vi "Traffic Control Project with Some more features.vi"() -> ()   [LabVIEW 2019]
uses:
  <vilib>/LabVIEW Interface for Arduino/Type Defs/Connection Type.ctl
  <vilib>/LabVIEW Interface for Arduino/Type Defs/Pin Mode.ctl
  <vilib>/LabVIEW Interface for Arduino/Type Defs/Board Type.ctl
  <vilib>/LabVIEW Interface for Arduino/LabVIEW Interface for Arduino.lvlib
panel:
  out "Boolean 3":bool
  out "Boolean 2":bool
  out "Boolean":bool
  in  "milliseconds to wait 3":u32
  in  "milliseconds to wait 2":u32
  in  "milliseconds to wait":u32
  in  "stop":bool
  in  "VISA resource":refnum<visa-resource-name>
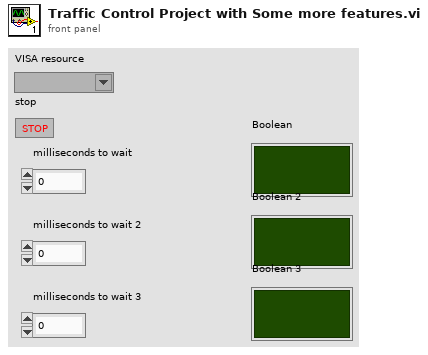
[diagram p1: front panel]
types:
  T1 = typedef "LabVIEW Interface for Arduino.lvlib/Board Type.ctl" = enum16{"Uno", "Dimuelanove w/Atmega 328", "Mega 2560"}
  T2 = typedef "LabVIEW Interface for Arduino.lvlib/Pin Mode.ctl" = enum8{"Input", "Output"}
  T3 = typedef "LabVIEW Interface for Arduino.lvlib/Connection Type.ctl" = enum8{"USB / Serial", "XBEE", "BlueSmirf (Bluetooth)"}
  T4 = typedef "LabVIEW Interface for Arduino.lvlib/Arduino Resource.ctl" = cluster{"VISA resource":refnum<visa-resource-name>, "Board Type":T1, "Connection Type":enum8{"USB / Serial"}, "Bytes Per Packet (15)":u8}
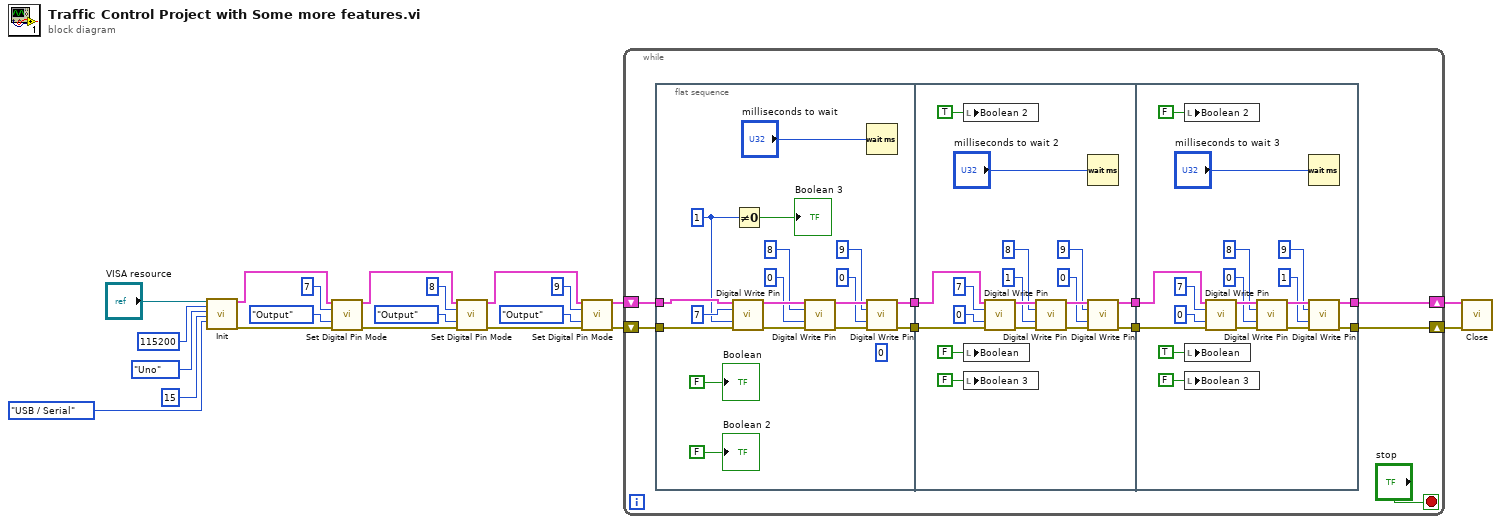
[diagram p0: block diagram]
diagram:
  n1 = call <vilib>:"Init.vi"("VISA resource"="VISA resource", "Baud Rate (115200)"=u32 115200, "Board Type (Uno)"=Board_Type."Uno", "Bytes Per Packet (15)"=u32 15, "Connection Type (USB/Serial)"=Connection_Type."USB / Serial") -> ("Arduino Resource"=w12:T4, "error out"=w13:errorcluster)  [unwired: 13 in]
  n2 = call <vilib>:"Set Digital Pin Mode.vi"("Arduino Resource"=w12, "Digital I/O Pin"=u8 7, "Pin Mode (Input)"=Pin_Mode."Output", "error in"=w13) -> ("Arduino Resource"=w17:T4, "error out"=w16:errorcluster)  [unwired: 10 in]
  n3 = call <vilib>:"Set Digital Pin Mode.vi"("Arduino Resource"=w17, "Digital I/O Pin"=u8 8, "Pin Mode (Input)"=Pin_Mode."Output", "error in"=w16) -> ("Arduino Resource"=w15:T4, "error out"=w14:errorcluster)  [unwired: 10 in]
  n4 = call <vilib>:"Set Digital Pin Mode.vi"("Arduino Resource"=w15, "Digital I/O Pin"=u8 9, "Pin Mode (Input)"=Pin_Mode."Output", "error in"=w14) -> ("Arduino Resource"=w5:T4, "error out"=w4:errorcluster)  [unwired: 10 in]
  n5 = while {
    shift-right: [w24] -> w3
    shift-left: w5 -> [w26]
    shift-right: [w23] -> w2
    shift-left: w4 -> [w25]
    stop <- "stop" stop-if-true
    n6 = flat-sequence {
      tunnel: w26 -> [w44]
      tunnel: w25 -> [w43]
      tunnel: [w39] -> w30
      tunnel: [w38] -> w29
      tunnel: w30 -> [w59]
      tunnel: w29 -> [w58]
      tunnel: [w57] -> w28
      tunnel: [w56] -> w27
      tunnel: w28 -> [w77]
      tunnel: w27 -> [w76]
      tunnel: [w72] -> w24
      tunnel: [w71] -> w23
      frame #0 {
        (unwired) u8 0 ("x")
        w32 = u8 1 ("Value (0)")
        n7 = call <vilib>:"Digital Write Pin.vi"("Arduino Resource"=w44, "Digital I/O Pin (0)"=u8 7, "Value (0)"=w32, "error in"=w43) -> ("Arduino Resource"=w48:T4, "error out"=w47:errorcluster)  [unwired: 10 in]
        n8 = Not Equal To 0?(x=w32) -> (x != 0?=→"Boolean 3":bool)
        n9 = call <vilib>:"Digital Write Pin.vi"("Arduino Resource"=w48, "Digital I/O Pin (0)"=u8 8, "Value (0)"=u8 0, "error in"=w47) -> ("Arduino Resource"=w46:T4, "error out"=w45:errorcluster)  [unwired: 10 in]
        n10 = Wait (ms)(milliseconds to wait="milliseconds to wait") -> ()  [unwired: 1 out]
        n11 = call <vilib>:"Digital Write Pin.vi"("Arduino Resource"=w46, "Digital I/O Pin (0)"=u8 9, "Value (0)"=u8 0, "error in"=w45) -> ("Arduino Resource"=w39:T4, "error out"=w38:errorcluster)  [unwired: 10 in]
        "Boolean 2" <- FALSE ("Boolean 2")
        "Boolean" <- FALSE ("Boolean")
      }
      frame #1 {
        n12 = local write "Boolean 2"(TRUE ("Boolean 2")) -> ()
        n13 = local write "Boolean"(FALSE ("Boolean")) -> ()
        n14 = local write "Boolean 3"(FALSE ("Boolean 3")) -> ()
        n15 = call <vilib>:"Digital Write Pin.vi"("Arduino Resource"=w59, "Digital I/O Pin (0)"=u8 7, "Value (0)"=u8 0, "error in"=w58) -> ("Arduino Resource"=w66:T4, "error out"=w65:errorcluster)  [unwired: 10 in]
        n16 = call <vilib>:"Digital Write Pin.vi"("Arduino Resource"=w66, "Digital I/O Pin (0)"=u8 8, "Value (0)"=u8 1, "error in"=w65) -> ("Arduino Resource"=w64:T4, "error out"=w63:errorcluster)  [unwired: 10 in]
        n17 = Wait (ms)(milliseconds to wait="milliseconds to wait 2") -> ()  [unwired: 1 out]
        n18 = call <vilib>:"Digital Write Pin.vi"("Arduino Resource"=w64, "Digital I/O Pin (0)"=u8 9, "Value (0)"=u8 0, "error in"=w63) -> ("Arduino Resource"=w57:T4, "error out"=w56:errorcluster)  [unwired: 10 in]
      }
      frame #2 {
        n19 = local write "Boolean 2"(FALSE ("Boolean 2")) -> ()
        n20 = local write "Boolean"(TRUE ("Boolean")) -> ()
        n21 = local write "Boolean 3"(FALSE ("Boolean 3")) -> ()
        n22 = call <vilib>:"Digital Write Pin.vi"("Arduino Resource"=w77, "Digital I/O Pin (0)"=u8 7, "Value (0)"=u8 0, "error in"=w76) -> ("Arduino Resource"=w84:T4, "error out"=w83:errorcluster)  [unwired: 10 in]
        n23 = call <vilib>:"Digital Write Pin.vi"("Arduino Resource"=w84, "Digital I/O Pin (0)"=u8 8, "Value (0)"=u8 0, "error in"=w83) -> ("Arduino Resource"=w82:T4, "error out"=w81:errorcluster)  [unwired: 10 in]
        n24 = Wait (ms)(milliseconds to wait="milliseconds to wait 3") -> ()  [unwired: 1 out]
        n25 = call <vilib>:"Digital Write Pin.vi"("Arduino Resource"=w82, "Digital I/O Pin (0)"=u8 9, "Value (0)"=u8 1, "error in"=w81) -> ("Arduino Resource"=w72:T4, "error out"=w71:errorcluster)  [unwired: 10 in]
      }
    }
  }
  n26 = call <vilib>:"Close.vi"("Arduino Resource"=w3, "error in"=w2) -> ()  [unwired: 13 in, 1 out]
